vi "ArrayLast_I.vi"(11 "1D Array In":i32[](array[numeric])) -> (0 "Last Element":i32, 1 "Head of Array":i32[](array[numeric]))   [LabVIEW 2013]
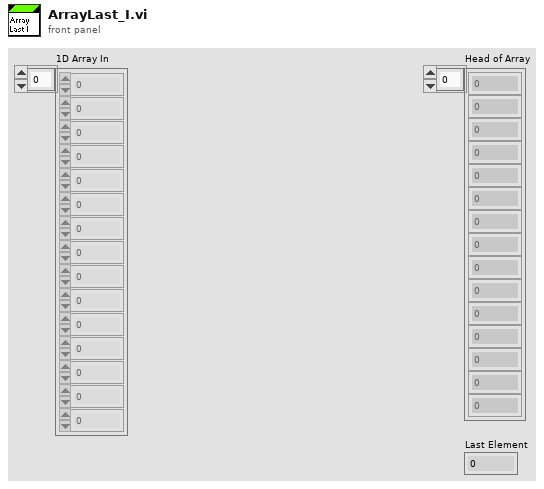
[diagram p1: front panel]
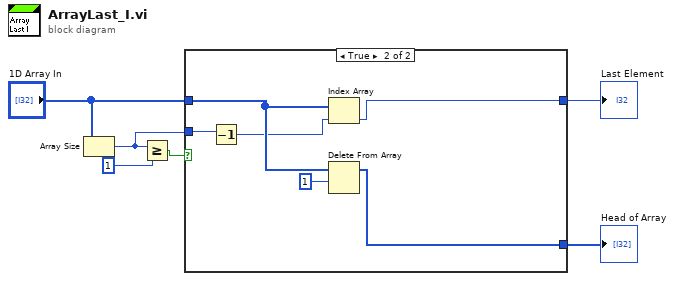
[diagram p0: block diagram]
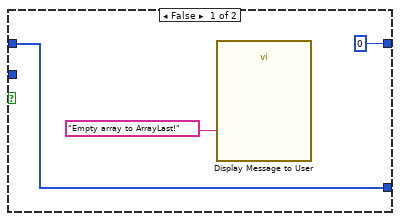
[diagram p2: hidden frame]
diagram:
  n1 = Array Size(array="1D Array In") -> (size(s)=w1:i32)
  n2 = Greater Or Equal?(x=w1, y=1) -> (x >= y?=w5:bool)
  n3 = case shown="True" w5 {
    tunnel: "1D Array In" -> [w8 w13]
    tunnel: [0 ("Numeric") w15] -> w3
    tunnel: [w8 w12] -> w2
    tunnel: w1 -> [_ w11]
    frame False {
      n4 = call "Display Message to User"("Message"="Empty array to ArrayLast!") -> ()  [unwired: 9 in, 2 out]
    }
    frame True {
      n5 = Decrement(x=w11) -> (x-1=w10:i32)
      n6 = Index Array(array=w13, index=w10) -> (element=w15:i32)
      n7 = Delete From Array(array=w13, length=1) -> (array with subset deleted=w12:i32[])  [unwired: 1 in, 1 out]
    }
  }
  "Last Element" <- w3
  "Head of Array" <- w2
